vi "Get LVObject.vi"(8 "error in (no error)":errorcluster, 11 "LVObjectMessage in":refnum<class "LVObjectMessage.lvclass">) -> (0 "error out":errorcluster, 2 "Message Data":refnum<class>, 3 "LVObjectMessage out":refnum<class "LVObjectMessage.lvclass">)   [LabVIEW 2009, in "LapDog.Messaging.v2.NativeTypes.lvlib" / "LVObjectMessage.lvclass"]
doc: "Returns the data contained in the message.\n\nThis method executes regardless of the error in state."
uses:
  LVObjectMessage.lvclass
  LVObjectMessage.lvclass/LVObjectMessage.ctl
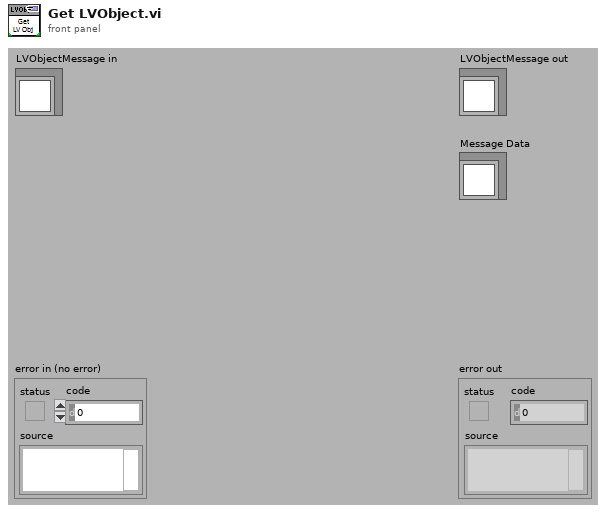
[diagram p1: front panel]
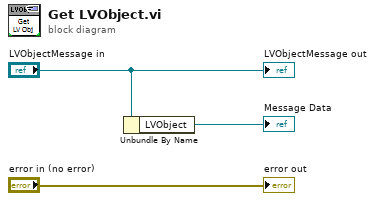
[diagram p0: block diagram]
diagram:
  n1 = Unbundle By Name("LVObjectMessage in") -> ("LVObject"=→"Message Data":refnum<class>)
  "error out" <- "error in (no error)"
  "LVObjectMessage out" <- "LVObjectMessage in"
